vi "CONEX-ALL Get Command Error String v2.vi"(7 "Error code":string, 9 "Connection Cluster in":T1) -> (1 "Error description":string, 3 "Connection Cluster out":T1)   [LabVIEW 2010]
doc: "Get description of error from error code.\n\nInput: Error Code\n\nOutput: Error Description matching code"
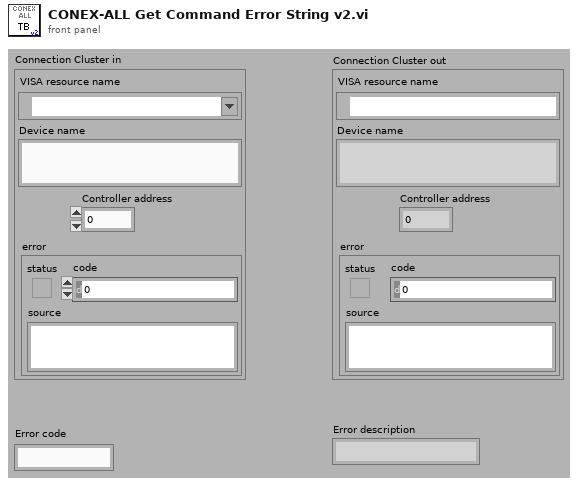
[diagram p1: front panel]
types:
  T1 = cluster{"VISA resource name":refnum<visa-resource-name>, "Device name":string, "Controller address":i32, "error":errorcluster}
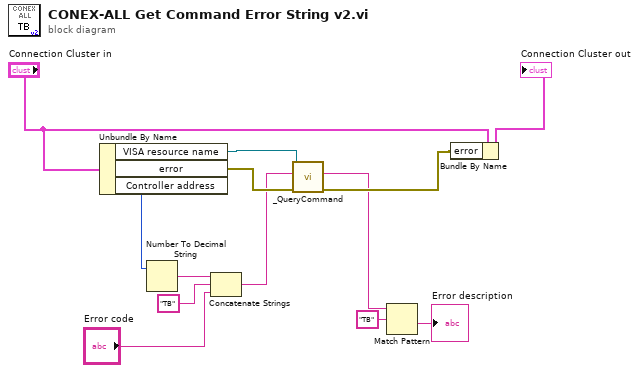
[diagram p0: block diagram]
diagram:
  n1 = Unbundle By Name("Connection Cluster in") -> ("VISA resource name"=w8:refnum<visa-resource-name>, "error"=w6:errorcluster, "Controller address"=w1:i32)
  n2 = Number To Decimal String(number=w1) -> (decimal integer string=w13:string)  [unwired: 1 out]
  n3 = Concatenate Strings(w13, "TB" ("strCommand"), "Error code") -> (w3:string)
  n4 = call <userlib>:"_QueryCommand.vi"("error in"=w6, "Command"=w3, "Instrument Channel in"=w8) -> ("error out"=w7:errorcluster, "Response"=w2:string)  [unwired: 6 in, 1 out]
  n5 = Match Pattern(string=w2, regular expression="TB" ("expression régulière")) -> (after substring=→"Error description":string)  [unwired: 4 out]
  n6 = Bundle By Name(cluster="Connection Cluster in", "error"=w7) -> (→"Connection Cluster out":T1)
